vi "GUI_resolutionSensitivity.vi"(8 "error in (no error)":errorcluster, 9 "resolution ref":refnum<vi>, 10 "sensitivity ref":refnum<vi>, 11 "Thorlabs_OSA300_64 in":refnum<class "OSA300.lvclass">) -> (0 "error out":errorcluster, 3 "Thorlabs_OSA300_64 out":refnum<class "OSA300.lvclass">)   [LabVIEW 2010, in "OSA300.lvclass"]
uses:
  OSA300.lvclass
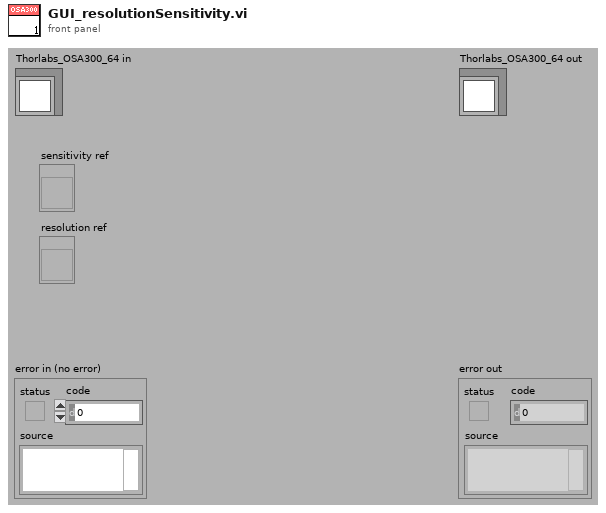
[diagram p1: front panel]
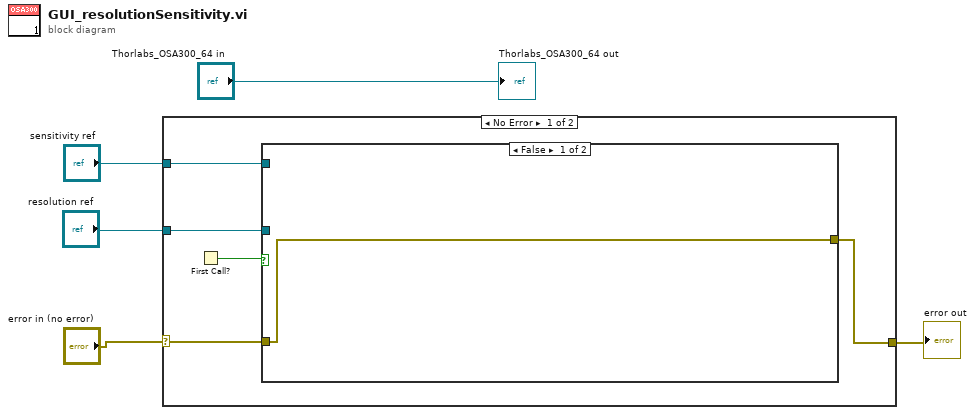
[diagram p0: block diagram]
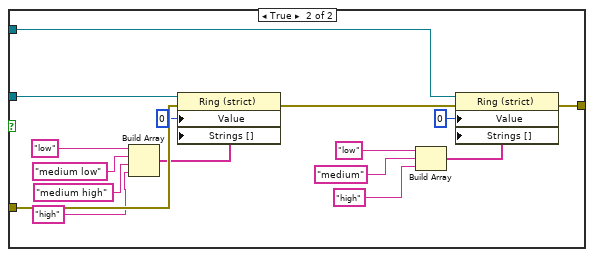
[diagram p2: hidden frame]
diagram:
  n1 = case shown="No Error" "error in (no error)" {
    selector: "error in (no error)" -> [w9 w28]
    tunnel: "resolution ref" -> [w10 _]
    tunnel: "sensitivity ref" -> [w8 _]
    tunnel: [w7 w28] -> w1
    frame No Error {
      n2 = First Call?() -> (First Call?: T/F=w6:bool)
      n3 = case shown="False" w6 {
        tunnel: w10 -> [_ w27]
        tunnel: w9 -> [w11 w25]
        tunnel: w8 -> [_ w24]
        tunnel: [w11 w17] -> w7
        frame False {
        }
        frame True {
          n4 = Build Array("low", "medium low", "medium high", "high") -> (w21:string[])
          n5 = property class="Ring (strict)"(reference=w27, error in=w25, "Value"=u16 0, "Strings []"=w21) -> (error out=w18:errorcluster)  [unwired: 1 out]
          n6 = Build Array("low", "medium", "high" ("element")) -> (w20:string[])
          n7 = property class="Ring (strict)"(reference=w24, error in=w18, "Value"=u16 0, "Strings []"=w20) -> (error out=w17:errorcluster)  [unwired: 1 out]
        }
      }
    }
    frame Error {
    }
  }
  "error out" <- w1
  "Thorlabs_OSA300_64 out" <- "Thorlabs_OSA300_64 in"
